vi "add_binary_data.vi"(4 "mime_type":string, 6 "filename":string, 8 "error in":errorcluster, 9 "data":u8[](array[numeric]), 10 "name":string, 11 "MultipartForm in":refnum<class "MultipartForm.lvclass">) -> (0 "error out":errorcluster, 2 "success":bool, 3 "MultipartForm out":refnum<class "MultipartForm.lvclass">)   [LabVIEW 2020, in "reqwest.lvlib" / "MultipartForm.lvclass"]
uses:
  MultipartForm.lvclass
  MultipartForm.lvclass/MultipartForm.ctl
  lv_reqwest_64.dll
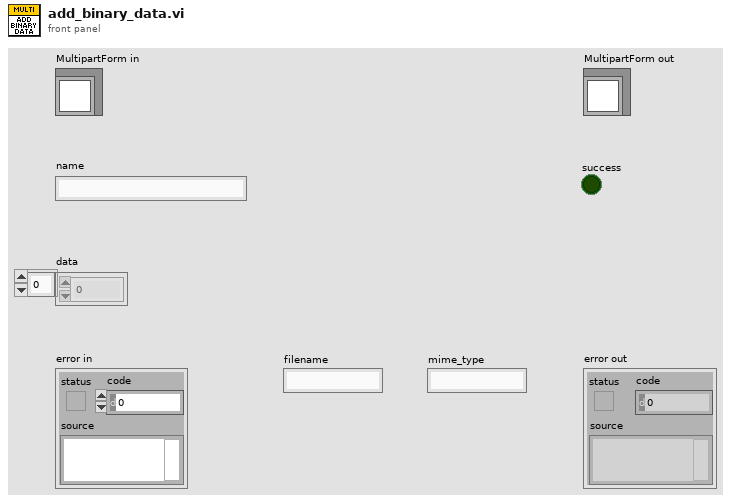
[diagram p1: front panel]
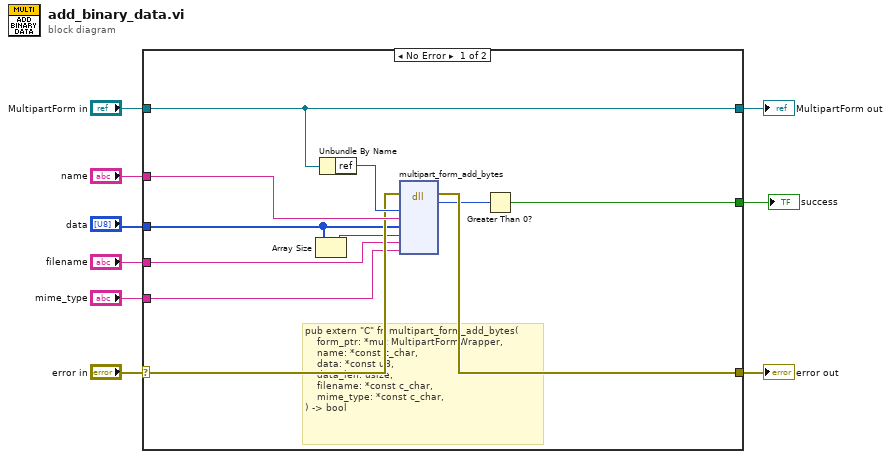
[diagram p0: block diagram]
diagram:
  n1 = case shown="No Error" "error in" {
    selector: "error in" -> [w17 w22]
    tunnel: [w16 w22] -> w8
    tunnel: [w20 w21] -> w6
    tunnel: "MultipartForm in" -> [w20 w21]
    tunnel: "name" -> [w18 _]
    tunnel: "data" -> [w13 _]
    tunnel: [w14 _] -> w3
    tunnel: "filename" -> [w11 _]
    tunnel: "mime_type" -> [w10 _]
    frame No Error {
      # "pub extern \"C\" fn multipart_form_add_bytes(\n    form_ptr: *mut MultipartFormWrapper,\n    name: *const c_char,\n    data: *const u8,\n    data_len: usize,\n    filename: *const c_char,\n    mime_type: *const c_char,\n) -> bool"
      n2 = Array Size(array=w13) -> (size(s)=w12:i32)
      n3 = Unbundle By Name(w20) -> ("ref"=w19:u64)
      n4 = dll-call lib="C:/Projects/reqwest-rs-labview/lv_src/lv_reqwest_*.*" fn="multipart_form_add_bytes"(error in=w17, "form_ptr"=w19, "name"=w18, "data"=w13, "data_len"=w12, "filename"=w11, "mime_type"=w10) -> (error out=w16:errorcluster, "bool"=w15:u8)  [unwired: 8 in, 1 out]
      n5 = Greater Than 0?(x=w15) -> (x > 0?=w14:bool)
    }
    frame Error {
    }
  }
  "error out" <- w8
  "MultipartForm out" <- w6
  "success" <- w3
